vi "Camera Manager Excute Command.vi"(8 "error in (no error)":errorcluster, 10 "Command":string, 11 "cameraId":i32) -> (0 "error out":errorcluster, 2 "Command out":string)   [LabVIEW 2017, in "PlayNitrideCameraComponet1010_4.lvlib"]
doc: "__declspec(dllexport) void CameraManager_ExcuteCommand(int cameraId, char* Command);"
uses:
  <userlib>/PlayNitrideCameraComponet1010_4/PlayNitrideCameraComponet1010_4.lvlib
  <userlib>/PlayNitrideCameraComponet1010_4/PlayNitrideCameraComponet.dll
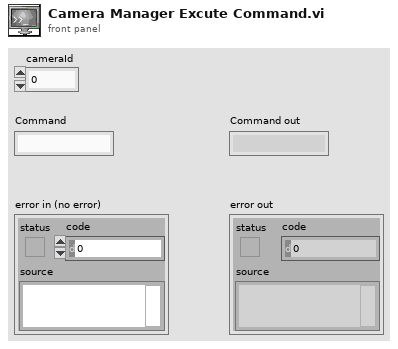
[diagram p1: front panel]
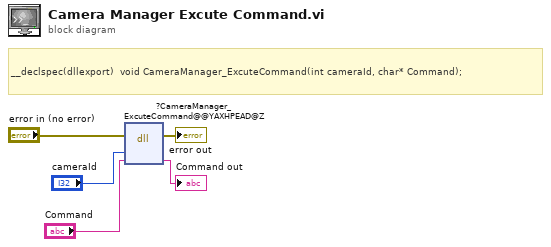
[diagram p0: block diagram]
diagram:
  # "__declspec(dllexport)  void CameraManager_ExcuteCommand(int cameraId, char* Command);"
  n1 = dll-call lib="C:/Program Files/National Instruments/LabVIEW 2017/user.lib/PlayNitrideCameraComponet1010_4/PlayNitrideCameraComponet.*" fn="?CameraManager_ExcuteCommand@@YAXHPEAD@Z"(error in="error in (no error)", "cameraId"="cameraId", "Command"="Command") -> (error out=→"error out":errorcluster, "Command"=→"Command out":string)  [unwired: 4 in, 1 out]
